vi "disabledUpdateList.vi"(8 "error in (no error)":errorcluster, 11 "Model in":refnum<class "Model.lvclass">) -> (0 "error out":errorcluster, 3 "Model out":refnum<class "Model.lvclass">)   [LabVIEW 2016, in "Model.lvclass"]
uses:
  Model.lvclass
  Model.lvclass/Model.ctl
  ILCCommunications/ILCCommunications.lvclass/ILCCommunications.ctl
  Common_RT_Modbus/ModbusBuffer/ModbusBuffer.lvclass/ModbusBuffer.ctl
  Common_RT_FAILC/FAILC/FAILC.lvclass/FAILC.ctl
  Common_RT_HPILC/HPILC/HPILC.lvclass/HPILC.ctl
  Common_RT_Modbus/ModbusBuffer/setIndex.vi
  ILCCommunications/broadcastFAFreezeSensorValues.vi
  ILCCommunications/broadcastHPFreezeSensorValues.vi
  Common_RT_FAILC/FAILC/addBroadcastFreezeSensorValuesFrame.vi
  Common_RT_HPILC/HPILC/addBroadcastFreezeSensorValuesFrame.vi
  Common_RT_Modbus/ModbusBuffer/writeHeader.vi
  Common_RT_Modbus/ModbusBuffer/writeU8.vi
  Common_RT_Modbus/ModbusBuffer/writeCRC.vi
  Common_RT_Modbus/ModbusBuffer/writeEndOfFrame.vi
  Common_RT_Modbus/ModbusBuffer/writeDelay.vi
  Common_RT_Modbus/ModbusBuffer/writeByteInstruction.vi
  Common_RT_Modbus/ModbusBuffer/calculateCRC.vi
  ILCCommunications/ILCCommunications.lvclass
  Resources/FPGA/FPGA.lvclass
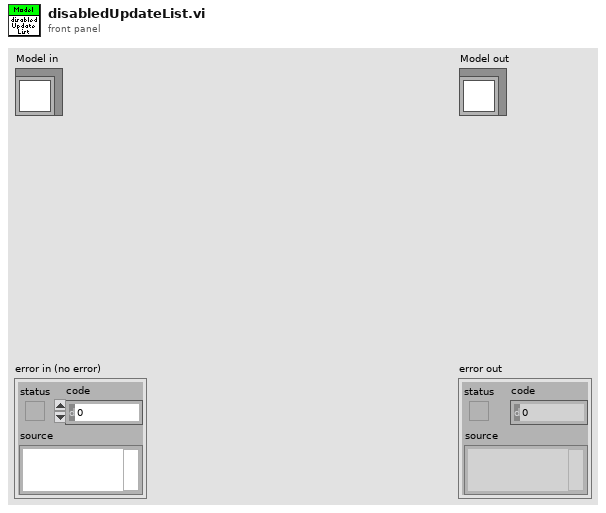
[diagram p1: front panel]
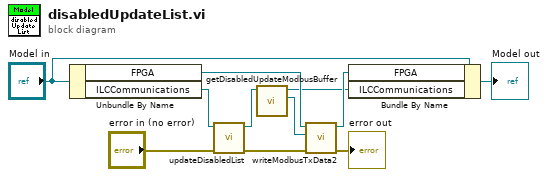
[diagram p0: block diagram]
diagram:
  n1 = Unbundle By Name("Model in") -> ("FPGA"=w9:refnum<class "FPGA.lvclass">, "ILCCommunications"=w11:refnum<class "ILCCommunications.lvclass">)
  n2 = call "updateDisabledList.vi"("error in (no error)"="error in (no error)", "ILCCommunications in"=w11) -> ("error out"=w7:errorcluster, "ILCCommunications out"=w10:refnum<class "ILCCommunications.lvclass">)  [unwired: 8 in]
  n3 = call "getDisabledUpdateModbusBuffer.vi"("ILCCommunications in"=w10) -> ("ModbusBuffer"=w8:refnum<class "ModbusBuffer.lvclass">, "ILCCommunications out"=w3:refnum<class "ILCCommunications.lvclass">)  [unwired: 9 in]
  n4 = call "writeModbusTxData2.vi"("error in (no error)"=w7, "ModbusBuffer in"=w8, "FPGA in"=w9) -> ("error out"=→"error out":errorcluster, "FPGA out"=w4:refnum<class "FPGA.lvclass">)  [unwired: 6 in, 1 out]
  n5 = Bundle By Name(cluster="Model in", "FPGA"=w4, "ILCCommunications"=w3) -> (→"Model out":refnum<class "Model.lvclass">)
